vi "DeviceClose.vi"(6 "Delay between send and receive [ms]":i32=100, 8 "error in (no error)":errorcluster, 11 "Monochromator in":refnum<class "Monochromator.lvclass">) -> (0 "error out":errorcluster, 1 "ID":i32, 2 "results-JSON string":string, 3 "Monochromator out":refnum<class "Monochromator.lvclass">, 4 "device is open?":bool)   [LabVIEW 2023, in "Monochromator.lvclass"]
doc: "Closes communications with the monochromator indicated by the index."
uses:
  Monochromator.lvclass
  GenericDevice/GenericDevice.lvclass
panel:
  # "Connector Pane"
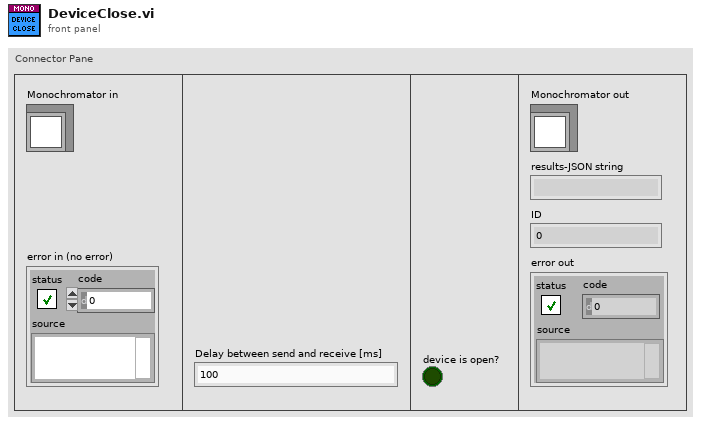
[diagram p1: front panel]
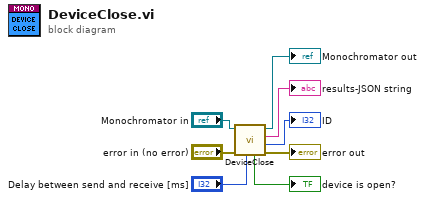
[diagram p0: block diagram]
diagram:
  n1 = call-parent "DeviceClose.vi"("Delay between send and receive [ms]"="Delay between send and receive [ms]", "error in (no error)"="error in (no error)", "GenericDevice in"="Monochromator in") -> ("error out"=→"error out":errorcluster, "ID"=→"ID":i32, "results-JSON string"=→"results-JSON string":string, "GenericDevice out"=→"Monochromator out":refnum<class "Monochromator.lvclass">, "device is open?"=→"device is open?":bool)  [unwired: 4 in]
